vi "Sort Fcurve Mdata_obj.vi"(0 "reference in":refnum<class "Fcurve.lvclass">, 5 "error in (no error)":errorcluster) -> (14 "reference out":refnum<class "Fcurve.lvclass">, 16 "Metadata out":T1, 19 "error out":errorcluster)   [LabVIEW 2019, in "Fcurve.lvclass"]
doc: "Sorts the Fcurve properties from the metadata input parameters"
uses:
  Fcurve.lvclass
  Metadata.ctl
  Loaded Fcurve parameters.ctl
  TDMS_DataHandler_class/PSnex TDMS fcurve property names.ctl
  metadata_class/metadata.lvclass
  TDMS_DataHandler_class/TDMS_DataHandler.lvclass
panel:
  out "1/x":dbl
  out "Array":string[](array[string])
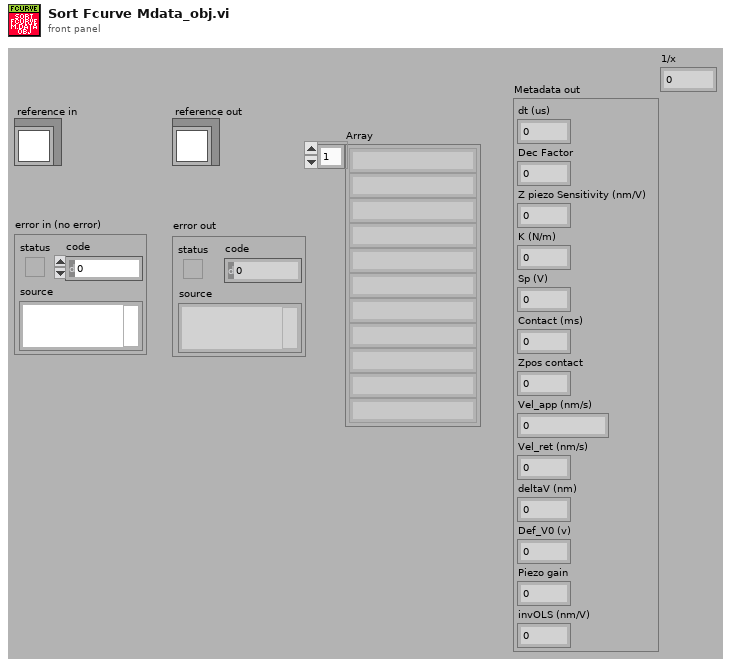
[diagram p1: front panel]
types:
  T1 = typedef "Fcurve.lvclass/Metadata.ctl" = cluster{"dt (us)":dbl, "Dec Factor":dbl, "Z piezo Sensitivity (nm/V)":dbl, "K (N/m)":dbl, "Sp (V)":dbl, "Contact (ms)":dbl, "Zpos contact":dbl, "Vel_app (nm/s)":dbl, "Vel_ret (nm/s)":dbl, "deltaV (nm)":dbl, "Def_V0 (v)":dbl, "Piezo gain":dbl, "invOLS (nm/V)":dbl}
  T2 = typedef "Fcurve.lvclass/Loaded Fcurve parameters.ctl" = T3[]
  T3 = typedef "TDMS_DataHandler.lvclass/PSnex TDMS fcurve property names.ctl" = string
  T4 = typedef "Fcurve.lvclass/ObjectAttributesRef.ctl" = refnum<data-value>
  T5 = typedef "Fcurve.lvclass/ObjectAttributes.ctl" = cluster{"MyAttribute":dbl, "Fcurve Metadata":T1, "Contact Spread of dev":dbl, "Tau Delay (ms)":dbl, "Points of contact":dbl, "Def_wfm":cluster{"Max":dbl, "Min":dbl}, "Zpos_wfm":cluster{"Max":dbl, "Min":dbl}, "Contact stat?":bool, "Real AI dt (s)":dbl, "Decimation":cluster{"App":cluster{"Dec":i32, "apply":bool}, "Con":cluster{"Dec":i32, "apply":bool}, "Ret":cluster{"Dec":i32, "apply":bool}}, "Segment def[0]":dbl, "Segment Zpos[0]":dbl, "Raw Datum":waveform(dbl)[], "Group metadata":T6, "M_data obj":refnum<class "metadata.lvclass">, "Channel name(s)":string[], "Segment fcurve data":cluster{"X":dbl[], "Y":dbl[]}[], "Segment duration":cluster{"Start":i32, "Duration":i32}[], "Segment info":T7[], "Segment durations (S)":dbl[], "Segments Maxmin":T9[]}
  T6 = typedef "TDMS_DataHandler.lvclass/Fcurve Meta data.ctl" = cluster{"property names":string[], "property values":variant[]}
  T7 = typedef "Fcurve.lvclass/Fcurve segments --cluster.ctl" = cluster{"type":T8, "nb points":i32, "dec factor":u32, "sampling rate (S/s)":u32}
  T8 = typedef "metadata.lvclass/Segment type--combobox.ctl" = string
  T9 = typedef "Fcurve.lvclass/Segment MaxMin --cluster.ctl" = cluster{"Def":cluster{"max value":dbl, "min value":dbl}, "Zpos":cluster{"max value":dbl, "min value":dbl}}
  T10 = typedef "metadata.lvclass/Fcurve segment.ctl" = cluster{"type":T8, "fast_fpga_trigger":bool, "nb":u8, "duration (ticks)":i64, "nb points":i32, "sampling rate (S/s)":u32, "Zpiezo control out":string, "initial deflection (V)":dbl, "relative setpoint":bool, "setpoint on":bool, "setpoint (V)":dbl, "setpoint trigger channel":string, "velocity (V/tick)":dbl, "Z position setpoint trigger (V)":dbl, "Z retract length (V)":dbl, "dec factor":u32}
  T11 = typedef "metadata.lvclass/XYZ piezos parameters.ctl" = cluster{"X stage piezo sensitivity (nm/V)":dbl, "X stage piezo gain":dbl, "X velocity (V/tick)":dbl, "X closed loop":bool, "Y stage piezo sensitivity (nm/V)":dbl, "Y stage piezo gain":dbl, "Y velocity (V/tick)":dbl, "Y closed loop":bool, "Z stage piezo sensitivity (nm/V)":dbl, "Z stage piezo gain":dbl, "Z closed loop":bool, "X position (V)":dbl, "Y position (V)":dbl}
  T12 = typedef "metadata.lvclass/Cantilever info parameters.ctl" = cluster{"spring constant calib method":string, "invOLS calib method":string, "thermal calib deflection channel":string, "model":string, "shape":string, "tip geometry":string, "Laser sum (V)":dbl, "Laser power (mA)":dbl, "invOLS_(nm/V)":dbl, "spring constant nominal (N/m)":dbl, "spring constant calib (N/m)":dbl, "resosnance frequency air calib (Hz)":dbl, "resosnance frequency calib (Hz)":dbl, "quality factor":dbl, "Acoefficident_GCI_(nN.s^1.3/m)":dbl, "half angle (deg)":dbl, "tip radius (m)":dbl, "tip height (m)":dbl, "system mount angle (deg)":dbl}
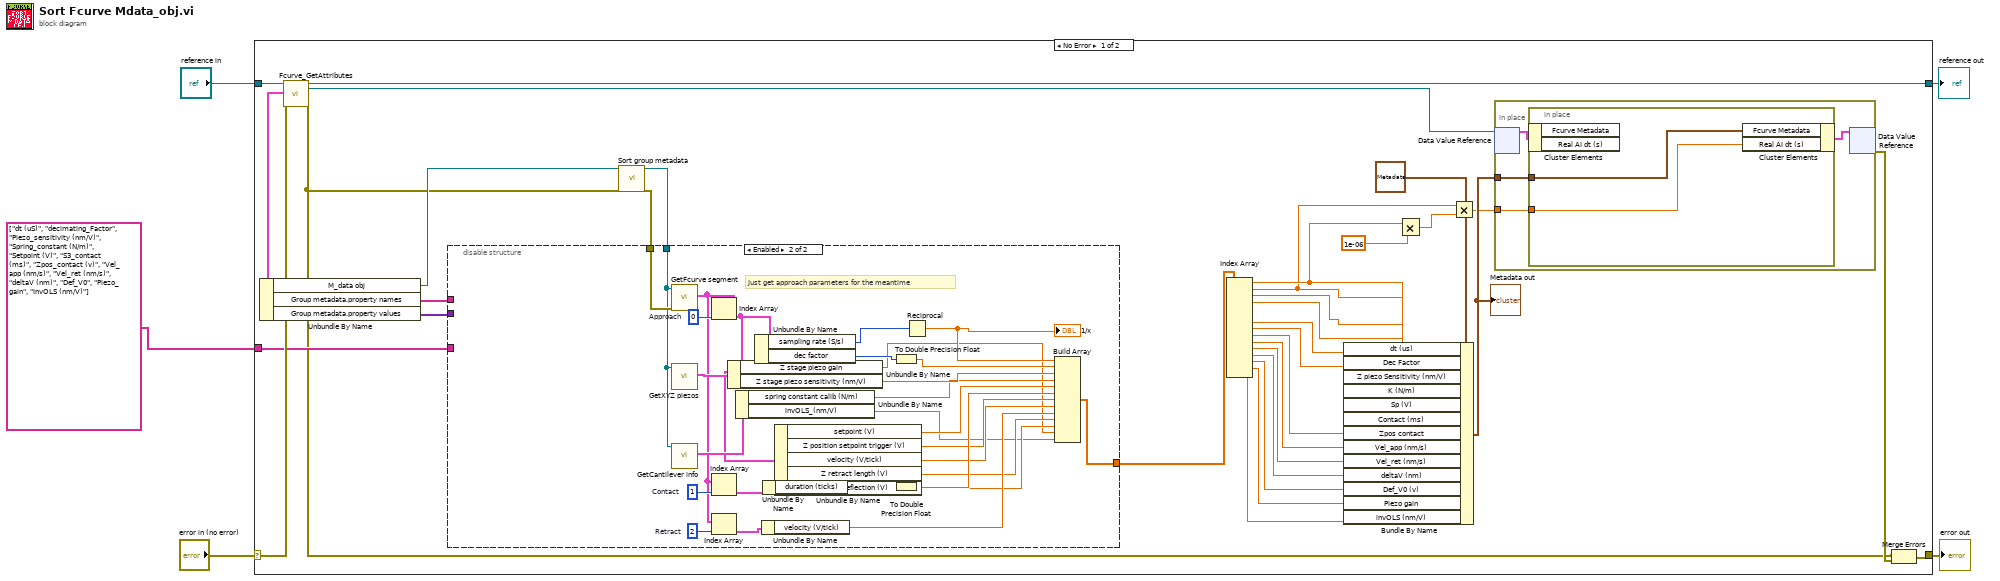
[diagram p0: block diagram]
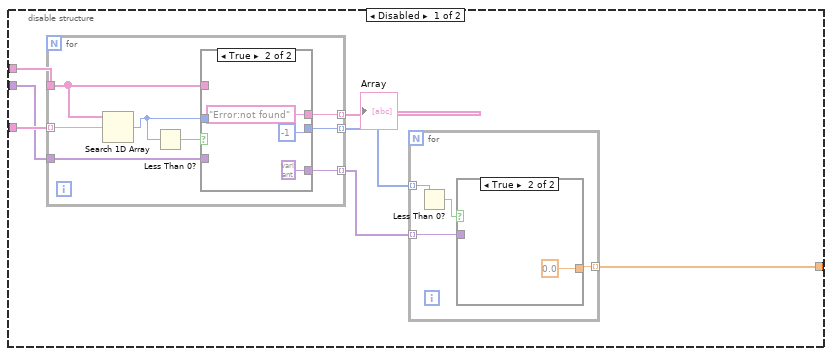
[diagram p2: hidden frame]
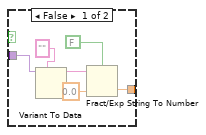
[diagram p3: hidden frame]
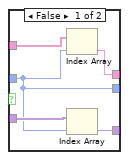
[diagram p4: hidden frame]
diagram:
  n1 = case shown="No Error" "error in (no error)" {
    selector: "error in (no error)" -> [w38 w108]
    tunnel: [w33 w108] -> w4
    tunnel: [w37 w107] -> w2
    tunnel: "reference in" -> [w35 w107]
    tunnel: T2 ["dt (uS)", "decimating_Factor", "Piezo_sensitivity (nm/V)", "Spring_constant (N/m)", "Setpoint (V)", "S3_contact (ms)", "Zpos_contact (v)", "Vel_app (nm/s)", "Vel_ret (nm/s)", "deltaV (nm)", "Def_V0", "Piezo_gain", "InvOLS (nm/V)"] ("Loaded Fcurve parameters") -> [w28 _]
    frame No Error {
      n2 = call "Fcurve_GetAttributes.vi"("reference in"=w35, "error in (no error)"=w38) -> ("reference out"=w37:refnum<class "Fcurve.lvclass">, "attributes ref"=w32:T4, "attributes"=w36:T5, "error out"=w8:errorcluster)  [unwired: 14 in]
      n3 = Unbundle By Name(w36) -> ("M_data obj"=w9:refnum<class "metadata.lvclass">, "Group metadata.property names"=w29:string[], "Group metadata.property values"=w27:variant[])
      n4 = call-dynamic "Sort group metadata.vi"("reference in"=w9, "error in (no error)"=w8) -> ("reference out"=w7:refnum<class "metadata.lvclass">, "error out"=w6:errorcluster)  [unwired: 16 in]
      n5 = disable-structure shown="Enabled" {
        disable-tunnel: w29 -> [w45 _]
        disable-tunnel: w28 -> [w44 _]
        disable-tunnel: w27 -> [w42 _]
        disable-tunnel: [w40 w97] -> w26
        disable-tunnel: w7 -> [_ w95]
        disable-tunnel: w6 -> [_ w100]
        frame Disabled {
          n6 = for {
            tunnel: w44 -> [w64] mode=indexing
            tunnel: [w63] -> w43 mode=indexing
            tunnel: w42 -> [w62]
            tunnel: [w60] -> w41 mode=indexing
            tunnel: [w58] -> w39 mode=indexing
            tunnel: w45 -> [w57]
            n7 = Search 1D Array(1D array=w57, element=w64) -> (index of element=w61:i32)  [unwired: 1 in]
            n8 = Less Than 0?(x=w61) -> (x < 0?=w59:bool)
            n9 = case shown="True" w59 {
              tunnel: [w66 "Error:not found"] -> w63
              tunnel: w62 -> [w69 _]
              tunnel: w61 -> [w65 _]
              tunnel: [w68 variant] -> w60
              tunnel: [w65 -1 ("index of element")] -> w58
              tunnel: w57 -> [w67 _]
              frame False {
                n10 = Index Array(array=w67, index=w65) -> (element=w66:string)
                n11 = Index Array(array=w69, index=w65) -> (element=w68:variant)
              }
              frame True {
              }
            }
          }
          "Array" <- w43
          n12 = for {
            tunnel: w41 -> [w49] mode=indexing
            tunnel: [w48] -> w40 mode=indexing
            tunnel: w39 -> [w47] mode=indexing
            n13 = Less Than 0?(x=w47) -> (x < 0?=w46:bool)
            n14 = case shown="True" w46 {
              tunnel: w49 -> [w55 _]
              tunnel: [w53 0.0] -> w48
              frame False {
                n15 = Variant To Data(type="", Variant=w55) -> (data=w50:string)  [unwired: 1 in, 1 out]
                n16 = Fract/Exp String To Number(use system decimal point (T)=FALSE, string=w50, default (0 dbl)=0.0 ("default (0 DBL)")) -> (number=w53:dbl)  [unwired: 1 in, 1 out]
              }
              frame True {
              }
            }
          }
        }
        frame Enabled {
          w81 = 2  # Retract
          w83 = 0  # Approach
          w87 = 1  # Contact
          # "Just get approach parameters for the meantime"
          n17 = call-dynamic "GetFcurve segment.vi"("error in (no error)"=w100, "reference in"=w95) -> ("Fcurve segment"=w82:T10[])  [unwired: 7 in, 2 out]
          n18 = call-dynamic "GetXYZ piezos.vi"("reference in"=w95) -> ("XYZ piezos"=w94:T11)  [unwired: 8 in, 2 out]
          n19 = call-dynamic "GetCantilever info.vi"("reference in"=w95) -> ("Cantilever info"=w93:T12)  [unwired: 8 in, 2 out]
          n20 = Index Array(array=w82, index=w83) -> (element=w89:T10)
          n21 = Index Array(array=w82, index=w87) -> (element=w86:T10)
          n22 = Index Array(array=w82, index=w81) -> (element=w78:T10)
          n23 = Unbundle By Name(w94) -> ("Z stage piezo gain"=w74:dbl, "Z stage piezo sensitivity (nm/V)"=w91:dbl)
          n24 = Unbundle By Name(w93) -> ("spring constant calib (N/m)"=w90:dbl, "invOLS_(nm/V)"=w73:dbl)
          n25 = Unbundle By Name(w89) -> ("sampling rate (S/s)"=w99:u32, "dec factor"=w96:u32)
          n26 = Unbundle By Name(w78) -> ("velocity (V/tick)"=w77:dbl)
          n27 = Unbundle By Name(w86) -> ("duration (ticks)"=w85:i64)
          n28 = Unbundle By Name(w89) -> ("setpoint (V)"=w88:dbl, "Z position setpoint trigger (V)"=w80:dbl, "velocity (V/tick)"=w79:dbl, "Z retract length (V)"=w76:dbl, "initial deflection (V)"=w75:dbl)
          n29 = To Double Precision Float(number=w96) -> (double precision float=w92:dbl)
          n30 = To Double Precision Float(number=w85) -> (double precision float=w84:dbl)
          n31 = Reciprocal(x=w99) -> (1/x=w98:dbl)
          "1/x" <- w98
          n32 = Build Array(w98, w92, w91, w90, w88, w84, w80, w79, w77, w76, w75, w74, w73) -> (w97:dbl[])
        }
      }
      n33 = Index Array(array=w26) -> (element #1=w12:dbl, element #2=w10:dbl, element #3=w25:dbl, element #4=w24:dbl, element #5=w23:dbl, element #6=w22:dbl, element #7=w21:dbl, element #8=w20:dbl, element #9=w19:dbl, element #10=w18:dbl, element #11=w17:dbl, element #12=w16:dbl, element #13=w15:dbl)  [unwired: 13 in]
      n34 = Bundle By Name(cluster=T1 {"dt (us)"=0.0, "Dec Factor"=0.0, "Z piezo Sensitivity (nm/V)"=0.0, "K (N/m)"=0.0, "Sp (V)"=0.0, "Contact (ms)"=0.0, "Zpos contact"=0.0, "Vel_app (nm/s)"=0.0, "Vel_ret (nm/s)"=0.0, "deltaV (nm)"=0.0, "Def_V0 (v)"=0.0, "Piezo gain"=0.0, "invOLS (nm/V)"=0.0} ("Fcurve Metadata"), "dt (us)"=w12, "Dec Factor"=w10, "Z piezo Sensitivity (nm/V)"=w25, "K (N/m)"=w24, "Sp (V)"=w23, "Contact (ms)"=w22, "Zpos contact"=w21, "Vel_app (nm/s)"=w20, "Vel_ret (nm/s)"=w19, "deltaV (nm)"=w18, "Def_V0 (v)"=w17, "Piezo gain"=w16, "invOLS (nm/V)"=w15) -> (w30:T1)
      "Metadata out" <- w30
      n35 = Multiply(x=w12, y=1e-06) -> (x*y=w13:dbl)
      n36 = Multiply(x=w10, y=w13) -> (x*y=w11:dbl)
      n37 = in-place {
        in-place-border: w30 -> [w102]
        in-place-border: w11 -> [w101]
        n38 = in-place-dvr #1(w32) -> (w103:T5)  [unwired: 1 out]
        n39 = in-place {
          in-place-border: w102 -> [w106]
          in-place-border: w101 -> [w105]
          n40 = in-place-cluster #2(w103) -> ()  [unwired: 2 out]
          n41 = in-place-cluster #2("Fcurve Metadata"=w106, "Real AI dt (s)"=w105) -> (w104:T5)
        }
        n42 = in-place-dvr #1(w104) -> (w34:errorcluster)  [unwired: 1 out]
      }
      n43 = Merge Errors(w8, w34) -> (w33:errorcluster)
    }
    frame Error {
    }
  }
  "error out" <- w4
  "reference out" <- w2
